vi "XmitMIMICCommand-2.vi"(6 "error in (no error)":errorcluster, 8 "Command array":u8[](array[numeric]) format="%x", 9 "ACK?":bool=TRUE) -> (0 "error out":errorcluster, 1 "ACK":bool, 2 "RecvBuff":string)   [LabVIEW 2014]
panel:
  out "MIMIC_CMD":string
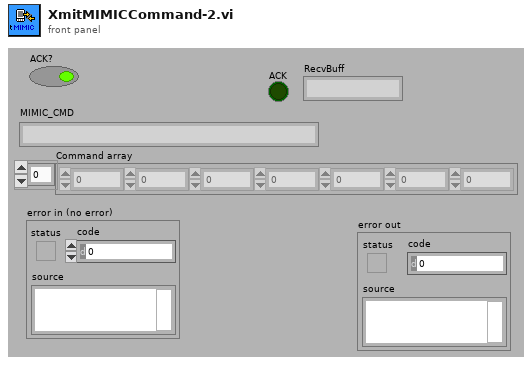
[diagram p1: front panel]
types:
  T1 = enum16{"OpenPort", "Initial Serial Port", "Write", "ByteRead", "Read", "ClearBuff", "Close"}
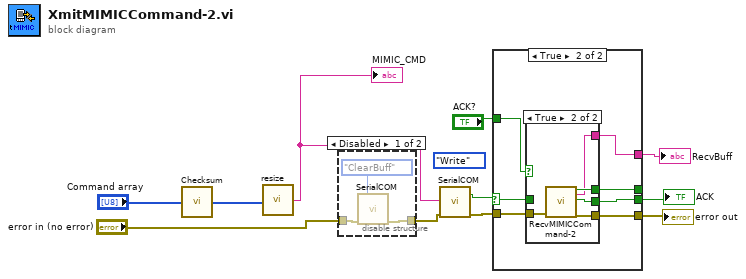
[diagram p0: block diagram]
diagram:
  (unwired) T1."Write" ("Function")
  n1 = call "Checksum.vi"("input array"="Command array") -> ("output array"=w10:u8[])
  n2 = call "resize.vi"("Array"=w10) -> ("MIMIC_CMD"=w9:string)
  "MIMIC_CMD" <- w9
  n3 = disable-structure shown="Disabled" {
    disable-tunnel: "error in (no error)" -> [w14 _]
    disable-tunnel: [w13 _] -> w7
    frame Disabled {
      n4 = call "SerialCOM.vi"("Function"=T1."ClearBuff", "error in (no error)"=w14) -> ("error out"=w13:errorcluster)  [unwired: 8 in, 5 out]
    }
    frame Enabled {
    }
  }
  n5 = call "SerialCOM.vi"("write buffer"=w9, "error in (no error)"=w7) -> ("Success?"=w4:bool, "error out"=w6:errorcluster)  [unwired: 8 in, 4 out]
  n6 = case shown="True" w4 {
    selector: w4 -> [w15 w17]
    tunnel: w6 -> [w16 w23]
    tunnel: [w16 w22] -> w5
    tunnel: [w15 w21] -> _
    tunnel: [w15 w20] -> w3
    tunnel: [_ w19] -> w2
    tunnel: "ACK?" -> [_ w18]
    frame False {
    }
    frame True {
      n7 = case shown="True" w18 {
        selector: w18 -> [w24 _]
        tunnel: w23 -> [w26 w31]
        tunnel: [w26 w30] -> w22
        tunnel: [w25 w29] -> w21
        tunnel: [w24 w28] -> w20
        tunnel: [_ w27] -> w19
        tunnel: w17 -> [w25 _]
        frame False {
        }
        frame True {
          n8 = call "RecvMIMICCommand-2.vi"("error in"=w31) -> ("success?"=w29:bool, "RecvBuff"=w27:string, "ACK"=w28:bool, "error out"=w30:errorcluster)  [unwired: 14 in, 1 out]
        }
      }
    }
  }
  "error out" <- w5
  "ACK" <- w3
  "RecvBuff" <- w2
